vi "Player Info.vi"(11 "Swirl in":refnum<class "Swirl.lvclass">) -> (0 "Defeat Speech":string, 1 "Victory Speech":string, 2 "Name":string, 3 "Swirl out":refnum<class "Swirl.lvclass">)   [LabVIEW 2015, in "Swirl.lvclass"]
uses:
  Swirl.lvclass
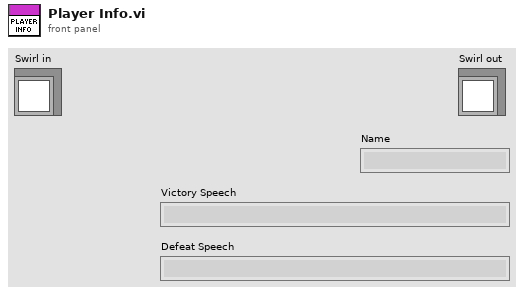
[diagram p1: front panel]
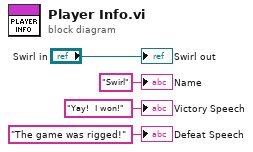
[diagram p0: block diagram]
diagram:
  "Swirl out" <- "Swirl in"
  "Name" <- "Swirl" ("Name")
  "Victory Speech" <- "Yay!  I won!" ("Victory Speech")
  "Defeat Speech" <- "The game was rigged!" ("Defeat Speech")
